vi "Main - Elapse to Sqrt Minutes (SubVI).vi"(11 "Elapse":string) -> (2 "sqrt (Minute)":dbl, 3 "Minute":dbl)   [LabVIEW 2019]
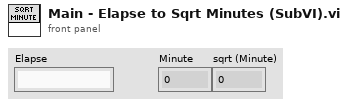
[diagram p1: front panel]
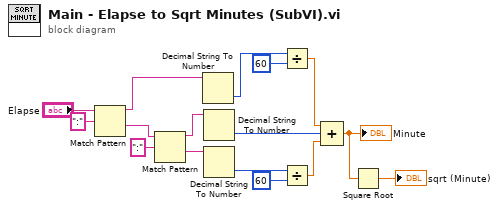
[diagram p0: block diagram]
diagram:
  n1 = Match Pattern(string="Elapse", regular expression=":") -> (before substring=w13:string, after substring=w14:string)  [unwired: 1 in, 2 out]
  n2 = Match Pattern(string=w14, regular expression=":") -> (before substring=w12:string, after substring=w11:string)  [unwired: 1 in, 2 out]
  n3 = Decimal String To Number(string=w13) -> (number=w10:i32)  [unwired: 2 in, 1 out]
  n4 = Decimal String To Number(string=w12) -> (number=w5:i32)  [unwired: 2 in, 1 out]
  n5 = Decimal String To Number(string=w11) -> (number=w7:i32)  [unwired: 2 in, 1 out]
  n6 = Divide(x=w10, y=60) -> (x/y=w6:dbl)
  n7 = Divide(x=w7, y=60) -> (x/y=w4:dbl)
  n8 = Compound Arithmetic op=ADD(w6, w5, w4) -> (w3:dbl)
  "Minute" <- w3
  n9 = Square Root(x=w3) -> (sqrt(x)=→"sqrt (Minute)":dbl)
